vi "Sequence.Test.DMC.GetComponentSize.vi"(9 "Component":T7, 10 "Plate":T1, 11 "OrderSets":T2={"State"=enum."Init", "ImgPath"=path "", "WabcoPlate"="", "WabcoProduct"="", "ClientProduct"="", "ClientPlate"="", "TotalQuantity"=0, "Serial"=0, "Wabco"={"LaserJob"="", "AdditionalTxt"="037", "FactoryCode"="", "RevID"=0, "ForkID"=0, "FailuresLimit"=0, "GlobalCnt"=0, "CheckDM"=FALSE, "SerialFormat"=enum."000001 - 499999", "CoordA"={"X"=0.0, "Y"=0.0, "Angle"=0.0}, "CoordB"={"X"=0.0, "Y"=0.0, "Angle"=0.0}, "DMCconfig"=0}, "Client"={"LaserJob"="", "AdditionalTxt"="", "FactoryCode"="037", "RevID"=0, "ForkID"=0, "FailuresLimit"=0, "GlobalCnt"=0, "CheckDM"=FALSE, "SerialFormat"=enum."000001 - 499999", "CoordA"={"X"=0.0, "Y"=0.0, "Angle"=0.0}, "CoordB"={"X"=0.0, "Y"=0.0, "Angle"=0.0}, "DMCconfig"=0}}) -> (1 "max size":i32, 2 "size":i32, 3 "Value":string)   [LabVIEW 2015]
uses:
  Gui/DMCConfiguatorGui.Component.ctl
  Gui/DMCConfiguatorGui.Type.ctl
  Gui/DMCConfiguatorGui.Var.ctl
  Logger/Logger.Variant.Sets.ctl
  Station/Station.Changeover.State.vi
  Station/Station.Plate.Properties.ctl
  Sequence.Code.SerialFormat.ctl
  Drivers/V7310/LowLevel/V7310.Job.Sets.ctl
  Sequence.PlateType.ctl
  Drivers/V7310/LowLevel/V7310.Global.vi
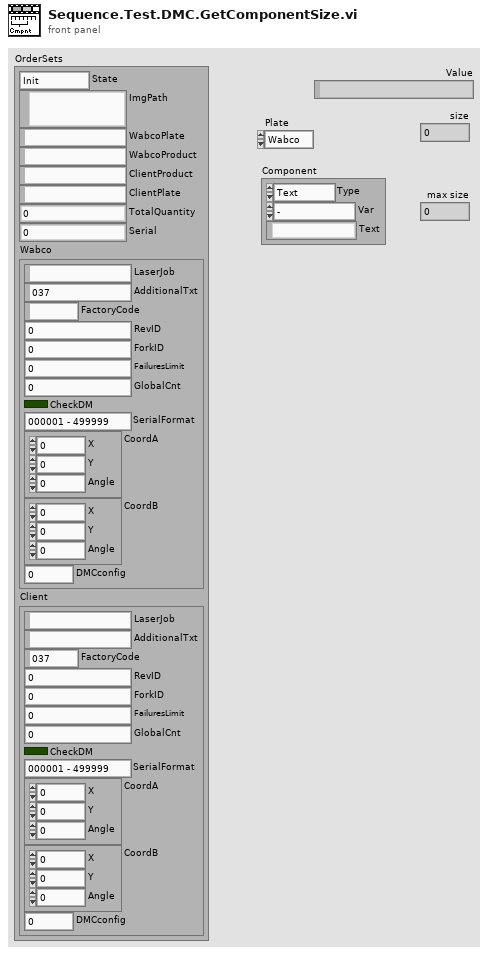
[diagram p1: front panel]
types:
  T1 = typedef "Sequence.PlateType.ctl" = enum16{"Wabco", "Client"}
  T2 = typedef "Logger.Variant.Sets.ctl" = cluster{"State":T3, "ImgPath":path, "WabcoPlate":string, "WabcoProduct":string, "ClientProduct":string, "ClientPlate":string, "TotalQuantity":u16, "Serial":i32, "Wabco":T4, "Client":T4}
  T3 = typedef "Station.Changeover.State.vi" = enum16{"Init", "Scaning", "NOK", "Wait for ack", "Ready"}
  T4 = typedef "Station.Plate.Properties.ctl" = cluster{"LaserJob":string, "AdditionalTxt":string, "FactoryCode":string, "RevID":u8, "ForkID":u8, "FailuresLimit":u16, "GlobalCnt":i32, "CheckDM":bool, "SerialFormat":T5, "CoordA":T6, "CoordB":T6, "DMCconfig":i32}
  T5 = typedef "Sequence.Code.SerialFormat.ctl" = enum8{"", "000001 - 499999", "500001 - 999999", "0000001 - 4999999", "5000001 - 9999999"}
  T6 = typedef "V7310.Job.Sets.ctl" = cluster{"X":dbl, "Y":dbl, "Angle":dbl}
  T7 = typedef "DMCConfiguatorGui.Component.ctl" = cluster{"Type":T8, "Var":T9, "Text":string}
  T8 = typedef "DMCConfiguatorGui.Type.ctl" = enum8{"Text", "Variable"}
  T9 = typedef "DMCConfiguatorGui.Var.ctl" = enum8{"-", "Wabco No", "Client No", "Serial", "Date"}
  T10 = typedef "V7310.Data.Status.ctl" = cluster{"State":T11, "LaserStatus":T12, "LaserStatusRaw":string, "Ref":refnum<k5>, "RTC TS":timestamp, "Conn TS":timestamp, "Msg":T13[], "JobInUse":string, "Jobs":string[], "Vars":T14[]}
  T11 = typedef "V7310.Data.Status.State.ctl" = enum16{"First", "Init", "Msg", "Error", "Abort", "Idle", "Run"}
  T12 = typedef "V7310.LaserStatus.ctl" = enum16{"-", "FatalError", "Initialize", "KeySwitchOpen", "TimeoutInterlock", "InterlockOpen", "StartUp", "ShutterlockOpen", "Standby", "Ready", "PrepareForMarking", "WaitForTrigger", "Marking"}
  T13 = typedef "V7310.Message.Data.ctl" = cluster{"ID":i32, "Msg":string}
  T14 = typedef "V7310.Job.Variable.ctl" = cluster{"Name":string, "Value":string}
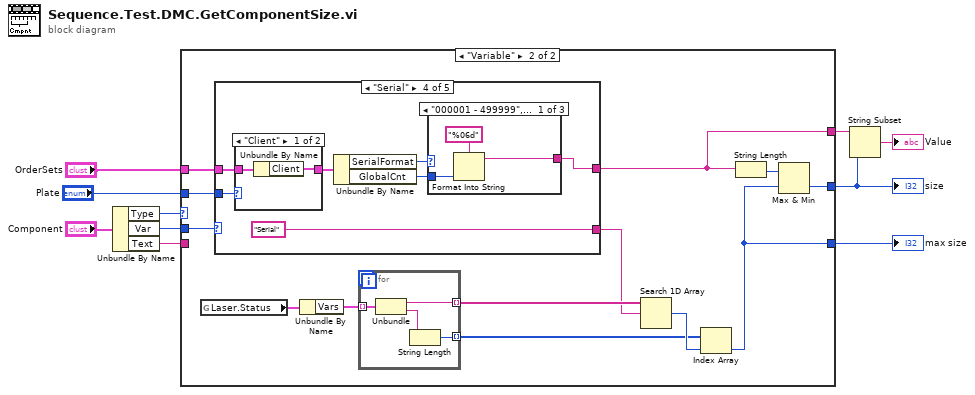
[diagram p0: block diagram]
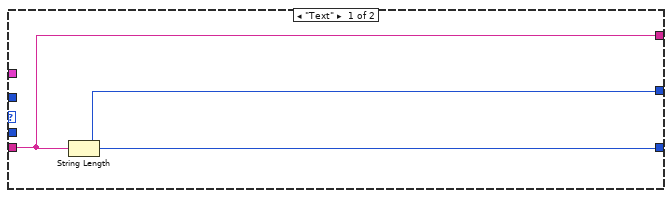
[diagram p2: hidden frame]
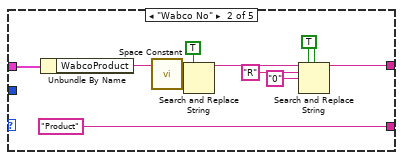
[diagram p4: hidden frame]
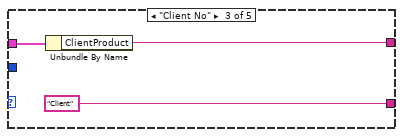
[diagram p5: hidden frame]
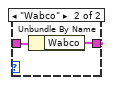
[diagram p6: hidden frame]
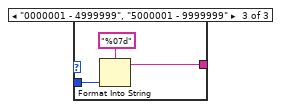
[diagram p8: hidden frame]
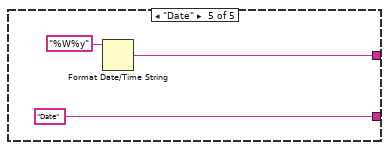
[diagram p9: hidden frame]
diagram:
  n1 = Unbundle By Name("Component") -> ("Type"=w9:T8, "Var"=w7:T9, "Text"=w8:string)
  n2 = case shown="\"Variable\"" w9 {
    tunnel: w8 -> [w11 _]
    tunnel: w7 -> [_ w20]
    tunnel: [w12 w15] -> w6
    tunnel: "OrderSets" -> [_ w18]
    tunnel: [w12 w13] -> w2
    tunnel: "Plate" -> [_ w17]
    tunnel: [w11 w14] -> w3
    frame "Text" {
      n3 = String Length(string=w11) -> (length=w12:i32)
    }
    frame "Variable" {
      n4 = global read "V7310.Global.vi" "Laser.Status"() -> (w25:T10)
      n5 = case shown="\"Serial\"" w20 {
        tunnel: [_ "Product" ("element") "Client" ("element") "Serial" ("element") "Date" ("element")] -> w19
        tunnel: w18 -> [_ w31 w37 w44 _]
        tunnel: [_ w26 w36 w39 w57] -> w14
        tunnel: w17 -> [_ _ _ w40 _]
        frame "-" {
        }
        frame "Wabco No" {
          w28 = TRUE ("replace all? (F)")
          n6 = Unbundle By Name(w31) -> ("WabcoProduct"=w32:string)
          n7 = call <vilib>:"Space Constant.vi"() -> ("String"=w34:string)
          n8 = Search and Replace String(replace all?=TRUE ("replace all? (F)"), input string=w32, search string=w34) -> (result string=w27:string)  [unwired: 5 in, 3 out]
          n9 = Search and Replace String(replace all?=w28, case sensitive?=w28, input string=w27, search string="R", replace string="0" ("replace string (\"\")")) -> (result string=w26:string)  [unwired: 3 in, 3 out]
        }
        frame "Client No" {
          n10 = Unbundle By Name(w37) -> ("ClientProduct"=w36:string)
        }
        frame "Serial" {
          n11 = case shown="\"Client\"" w40 {
            tunnel: w44 -> [w47 w49]
            tunnel: [w46 w48] -> w43
            frame "Client" {
              n12 = Unbundle By Name(w47) -> ("Client"=w46:T4)
            }
            frame "Wabco" {
              n13 = Unbundle By Name(w49) -> ("Wabco"=w48:T4)
            }
          }
          n14 = Unbundle By Name(w43) -> ("SerialFormat"=w42:T5, "GlobalCnt"=w41:i32)
          n15 = case shown="\"000001 - 499999\", \"500001 - 999999\"" w42 {
            tunnel: w41 -> [w52 _ w55]
            tunnel: [w50 _ w53] -> w39
            frame "000001 - 499999", "500001 - 999999" {
              n16 = Format Into String(format string="%06d", w52) -> (resulting string=w50:string)  [unwired: 2 in, 1 out]
            }
            frame "" {
            }
            frame "0000001 - 4999999", "5000001 - 9999999" {
              n17 = Format Into String(format string="%07d", w55) -> (resulting string=w53:string)  [unwired: 2 in, 1 out]
            }
          }
        }
        frame "Date" {
          n18 = Format Date/Time String(time format string (%c)="%W%y") -> (date/time string=w57:string)  [unwired: 2 in]
        }
      }
      n19 = Unbundle By Name(w25) -> ("Vars"=w24:T14[])
      n20 = for {
        tunnel: w24 -> [w62] mode=indexing
        tunnel: [w61] -> w22 mode=indexing
        tunnel: [w59] -> w21 mode=indexing
        n21 = Unbundle(w62) -> ("Name"=w61:string, "Value"=w60:string)
        n22 = String Length(string=w60) -> (length=w59:i32)
      }
      n23 = Search 1D Array(1D array=w22, element=w19) -> (index of element=w23:i32)  [unwired: 1 in]
      n24 = Index Array(array=w21, index=w23) -> (element=w15:i32)
      n25 = String Length(string=w14) -> (length=w16:i32)
      n26 = Max & Min(x=w16, y=w15) -> (min(x,y)=w13:i32)  [unwired: 1 out]
    }
  }
  "max size" <- w6
  "size" <- w2
  n27 = String Subset(string=w3, length (rest)=w2) -> (substring=→"Value":string)  [unwired: 1 in]
